vi "Windows UI.vi"() -> ()   [LabVIEW 2016]
doc: "This is the primary host VI which reads and displays current value data from shared variables running on the target."
panel:
  out "Stage 3":bool
  out "Stage 2":bool
  out "Stage 1":bool
  in  "Stop UI":bool
  out "Amplitude":dbl format="%#_3g"
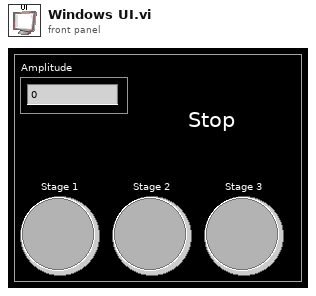
[diagram p1: front panel]
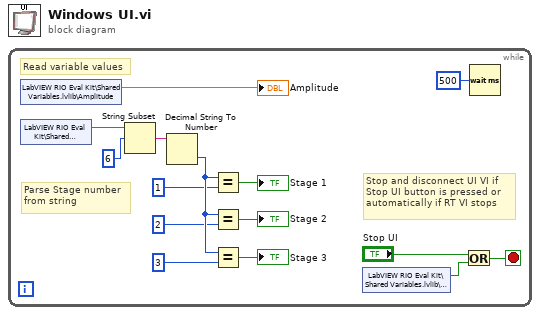
[diagram p0: block diagram]
diagram:
  n1 = while {
    stop <- w12 stop-if-true
    # "Stop and disconnect UI VI if \nStop UI button is pressed or \nautomatically if RT VI stops"
    # "Parse Stage number\nfrom string"
    # "Read variable values"
    n2 = shared-variable "LabVIEW RIO Eval Kit\\Shared Variables.lvlib\\Amplitude"() -> (→"Amplitude":dbl)  [unwired: 1 in, 1 out]
    n3 = shared-variable "LabVIEW RIO Eval Kit\\Shared Variables.lvlib\\State"() -> (w7:string)  [unwired: 1 in, 1 out]
    n4 = String Subset(string=w7, offset (0)=6) -> (substring=w5:string)  [unwired: 1 in]
    n5 = Decimal String To Number(string=w5) -> (number=w4:i32)  [unwired: 2 in, 1 out]
    n6 = Equal?(x=w4, y=1 ("offset (0)")) -> (x = y?=→"Stage 1":bool)
    n7 = Equal?(x=w4, y=2 ("offset (0)")) -> (x = y?=→"Stage 2":bool)
    n8 = Equal?(x=w4, y=3 ("offset (0)")) -> (x = y?=→"Stage 3":bool)
    n9 = shared-variable "LabVIEW RIO Eval Kit\\Shared Variables.lvlib\\Stop UI?"() -> (w13:bool)  [unwired: 1 in, 1 out]
    n10 = Or(x="Stop UI", y=w13) -> (x .or. y?=w12:bool)
    n11 = Wait (ms)(milliseconds to wait=u32 500) -> ()  [unwired: 1 out]
  }
